vi "Handle Error.vi"(8 "error in (no error)":errorcluster, 11 "Controller Actor in":refnum<class "Controller Actor.lvclass">) -> (0 "error out":errorcluster, 2 "stop actor?":bool=TRUE, 3 "Controller Actor out":refnum<class "Controller Actor.lvclass">)   [LabVIEW 2023, in "Event Actors.lvlib" / "Controller Actor.lvclass"]
doc: "(<B>Filename</B>: Actor Framework.lvlib:Actor.lvclass:Handle Error.vi)\n\nDefines how the actor handles an error that occurred while processing a message. By default, this method does nothing except stop the actor."
uses:
  Controller Actor.lvclass
  <vilib>/ActorFramework/Actor/Actor.lvclass/Actor.ctl
  Hardware Controller/Source/IError Messages/Pass Error Msg/Pass Error Msg.lvclass/Pass Error Msg.ctl
  <vilib>/ActorFramework/Message Enqueuer/Message Enqueuer.lvclass/Message Enqueuer.ctl
  <vilib>/ActorFramework/Message Enqueuer/Enqueue.vi
  Hardware Controller/Source/IError Messages/Pass Error Msg/Pass Error Msg.lvclass
  <vilib>/Utility/LVClass/Get LV Class Name.vi
  <resource>/AFDebug/Generate Trace for Message.vi
  <vilib>/ActorFramework/Message Priority Queue/Priority Enqueue.vi
  Controller Actor.lvclass/Controller Actor.ctl
  <vilib>/ActorFramework/Actor/Actor.lvclass
  C:/Program Files/National Instruments/LabVIEW 2023/vi.lib/MGI/Monitored Actor/Monitored Actor/Monitored Actor/Monitored Actor.lvclass
  C:/Program Files/National Instruments/LabVIEW 2023/vi.lib/ActorFramework/Actor/Actor.lvclass
  C:/Projects/Shared Libraries/Event Actors/Controller Actor/Controller Actor.lvclass
  C:/Projects/Hardware Controller/Source/IError/IError.lvclass
  C:/Projects/Hardware Controller/Source/LSI Hardware Controller/View Interface/IView.lvclass
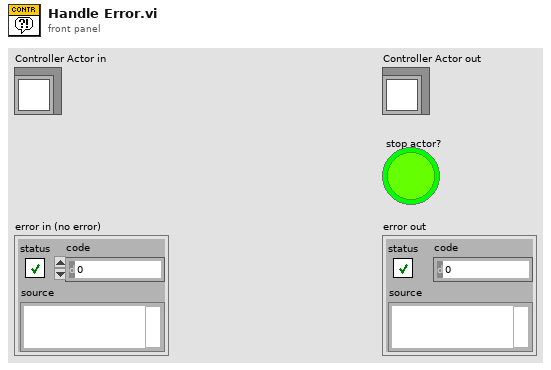
[diagram p1: front panel]
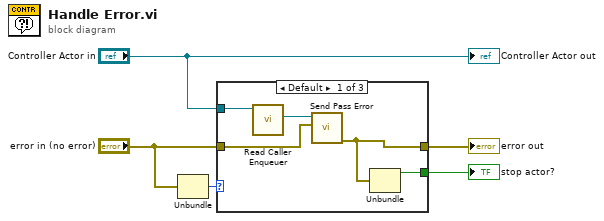
[diagram p0: block diagram]
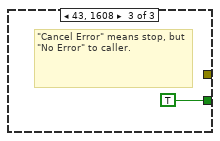
[diagram p3: hidden frame]
diagram:
  n1 = Unbundle("error in (no error)") -> ("code"=w5:i32)  [unwired: 2 out]
  n2 = case shown="Default" w5 {
    tunnel: [w8 _ _] -> w4
    tunnel: [w7 _ TRUE] -> w3
    tunnel: "Controller Actor in" -> [w10 _ _]
    tunnel: "error in (no error)" -> [w6 _ _]
    frame Default {
      n3 = call <vilib>:"Read Caller Enqueuer.vi"("Actor"=w10) -> ("Caller Enqueuer"=w9:refnum<class "Message Enqueuer.lvclass">)  [unwired: 10 in]
      n4 = call "Send Pass Error.vi"("error in"=w6, "Message Enqueuer"=w9) -> ("error out"=w8:errorcluster)  [unwired: 8 in, 1 out]
      n5 = Unbundle(w8) -> ("status"=w7:bool)  [unwired: 2 out]
    }
    frame 0 {
    }
    frame 43, 1608 {
      # "\"Cancel Error\" means stop, but \"No Error\" to caller."
    }
  }
  "error out" <- w4
  "stop actor?" <- w3
  "Controller Actor out" <- "Controller Actor in"
